vi "Standard Bus Write--SubVI.vi"(8 "error in":errorcluster, 9 "Set Value":string, 10 "Register":T1, 11 "Watlow F4T in":refnum<class "Watlow F4T.lvclass">) -> (0 "error out":errorcluster, 3 "Watlow F4T out":refnum<class "Watlow F4T.lvclass">)   [LabVIEW 2024, in "Watlow F4T.lvclass"]
uses:
  Watlow F4T.lvclass
  Controls/Standard Bus Register LUT Data--Cluster.ctl
  Watlow F4T.lvclass/Watlow F4T.ctl
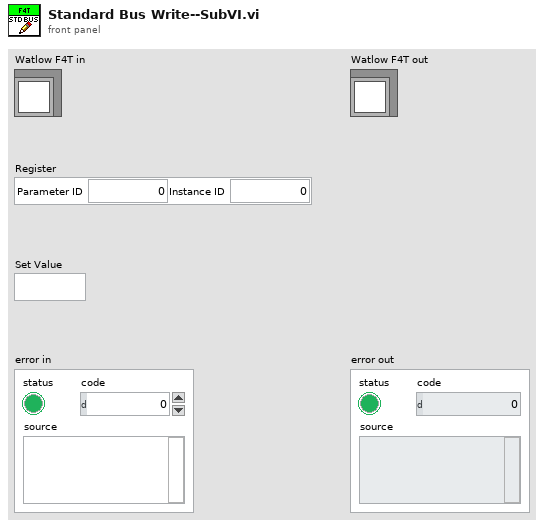
[diagram p1: front panel]
types:
  T1 = typedef "Watlow F4T.lvclass/Standard Bus Register LUT Data--Cluster.ctl" = cluster{"Parameter ID":i32, "Instance ID":i32}
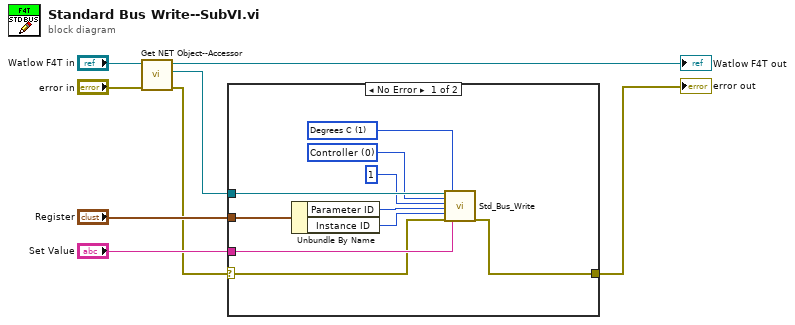
[diagram p0: block diagram]
diagram:
  n1 = call "Get NET Object--Accessor.vi"("error in (no error)"="error in", "Watlow F4T in"="Watlow F4T in") -> ("error out"=w4:errorcluster, ".NET Object"=w3:refnum<k24>, "Watlow F4T out"=→"Watlow F4T out":refnum<class "Watlow F4T.lvclass">)  [unwired: 7 in]
  n2 = case shown="No Error" w4 {
    selector: w4 -> [w15 w19]
    tunnel: w3 -> [w18 _]
    tunnel: "Set Value" -> [w17 _]
    tunnel: "Register" -> [w16 _]
    tunnel: [w14 w19] -> w2
    frame No Error {
      w9 = u8 1 items=["Degrees F", "Degrees C"] ("TemperatureUnits")
      w13 = 0 items=["Controller", "RUI", "PC", "CommsCard"] ("deviceType")
      n3 = Unbundle By Name(w16) -> ("Parameter ID"=w11:i32, "Instance ID"=w10:i32)
      n4 = call <instrlib>:"Std_Bus_Write.vi"("ILabVIEW In"=w18, "deviceType"=w13, "Zone"=1, "ParameterID"=w11, "InstanceId"=w10, "error in (no error)"=w15, "TemperatureUnits"=w9, "WriteValue"=w17) -> ("error out"=w14:errorcluster)  [unwired: 10 in, 1 out]
    }
    frame Error {
    }
  }
  "error out" <- w2
